vi "SaveTempData.vi"(2 "temp data":dbl[][][](array[numeric]), 3 "Exp_params":T3={"filename"="201612011532", "ExpFilePath"=path "\\\\10.0.0.7\\takada2/DATA/HBT6/data/Test/201612011532.h5", "File Ref list"=[16777216, 33554432], "sweep_dim"=[4, 2], "sweep_list"=[], "readout_list"=["ADC0", "ADC1"], "Sweep instrument bools"=[[0, 0], [0, 0], [0, 0], [0, 0], [0, 0], [0, 0], [0, 0], [0, 0], [0, 0], [0, 0], [0, 0], [0, 0], [0, 0], [0, 0], [0, 0], [0, 0], [0, 0], [0, 0], [0, 0], [0, 0], [0, 0], [0, 0], [0, 0], [0, 0], [0, 0], [0, 0], [0, 0], [0, 0], [0, 0], [0, 0], [0, 0]], "Read out instrument bools"=[[1, 0]], "Experimental bool list"=[FALSE, TRUE], "Initial move"=[{"Name"="None", "kind"=100, "Value"=0.0}], "FPGA Ref"=refnum, "Inst_parameters"={"ConfigFilePath"=path "\\\\10.0.0.7\\takada2/DATA/HBT6/data/Configs/HBT6_ramp_1.h5", "Inst_list"=["ADC", "AWG", "Freq", "Power", "sus", "rus", "rls", "sls", "suq", "suu", "sur", "suc", "sul", "ruq", "ruu", "rur", "ruc", "rul", "rlq", "rlu", "rlr", "rlc", "rll", "slq", "slu", "slr", "slc", "sll", "tu", "t", "tl", "fast_sequence"], "fast_mode"=[1, 1], "Wait_times"=[1, 1, 1, 1], "Inst_array"=[{"Kind"=0, "Strings"=["ADC", "", "V", "ADC0;ADC1", "V;V", "1.0;1.0"], "uint64s"=[10, 2, 250000, 0, 100, 10106, 1000000, 1, 0, 1], "Doubles"=[1.0], "DAQmx take out list"=[]}, {"Kind"=7, "Strings"=["AWG", "10.0.0.4", "", "C:\\Documents and Settings\\Bauerle\\Mes documents\\Bautze\\FPGA-clean_works_1.13.6_batchtest\\Python\\AWG", "dummy", "SAWnstrig_v4.py"], "uint64s"=[2, 0, 0, 3, 0, 0, 0, 0, 0, 0, 0, 0, 0, 0], "Doubles"=[1200000000.0, 1.0, 0.0, 1.0, 0.0, 1.0, 0.0, 1.0, 0.0, 1.0, 0.0, 1.0, 0.0], "DAQmx take out list"=[]}, {"Kind"=6, "Strings"=["Freq", "0:19", "GHz"], "uint64s"=[1, 0, 0, 0, 2, 0, 0, 0], "Doubles"=[2.0, -30.0, 200.0, 100.0, 0.0, 6.000999927520752, 9.000000318337698e-06, 30.0, -145.0], "DAQmx take out list"=[]}, {"Kind"=6, "Strings"=["Power", "0:19", "GHz"], "uint64s"=[1, 0, 1, 0, 2, 0, 0, 0], "Doubles"=[2.0, -30.0, 200.0, 100.0, 0.0, 6.000999927520752, 9.000000318337698e-06, 30.0, -145.0], "DAQmx take out list"=[]}, {"Kind"=4, "Strings"=["sus", "10.0.0.2", "mV"], "uint64s"=[0, 1], "Doubles"=[1.0, -1.0, 1.0, -1.0, 1.0], "DAQmx take out list"=[]}, {"Kind"=4, "Strings"=["rus", "10.0.0.2", "mV"], "uint64s"=[0, 2], "Doubles"=[1.0, -1.0, 1.0, -1.0, 1.0], "DAQmx take out list"=[]}, {"Kind"=4, "Strings"=["rls", "10.0.0.2", "mV"], "uint64s"=[0, 3], "Doubles"=[1.0, -1.0, 1.0, -1.0, 1.0], "DAQmx take out list"=[]}, {"Kind"=4, "Strings"=["sls", "10.0.0.2", "mV"], "uint64s"=[0, 4], "Doubles"=[1.0, -1.0, 1.0, -1.0, 1.0], "DAQmx take out list"=[]}, {"Kind"=4, "Strings"=["suq", "10.0.0.2", "V"], "uint64s"=[0, 5], "Doubles"=[0.30000001192092896, -2.0, 1.0, -1.0, 1.0], "DAQmx take out list"=[]}, {"Kind"=4, "Strings"=["suu", "10.0.0.2", "V"], "uint64s"=[0, 6], "Doubles"=[0.30000001192092896, -2.0, 1.0, -1.0, 1.0], "DAQmx take out list"=[]}, {"Kind"=4, "Strings"=["sur", "10.0.0.2", "V"], "uint64s"=[0, 7], "Doubles"=[0.30000001192092896, -2.0, 1.0, -1.0, 1.0], "DAQmx take out list"=[]}, {"Kind"=4, "Strings"=["suc", "10.0.0.2", "V"], "uint64s"=[1, 0], "Doubles"=[0.30000001192092896, -2.0, 1.0, -1.0, 1.0], "DAQmx take out list"=[]}, {"Kind"=4, "Strings"=["sul", "10.0.0.2", "V"], "uint64s"=[1, 1], "Doubles"=[0.30000001192092896, -2.0, 1.0, -1.0, 1.0], "DAQmx take out list"=[]}, {"Kind"=4, "Strings"=["ruq", "10.0.0.2", "V"], "uint64s"=[1, 2], "Doubles"=[0.30000001192092896, -2.0, 1.0, -1.0, 1.0], "DAQmx take out list"=[]}, {"Kind"=4, "Strings"=["ruu", "10.0.0.2", "V"], "uint64s"=[1, 3], "Doubles"=[0.30000001192092896, -2.0, 1.0, -1.0, 1.0], "DAQmx take out list"=[]}, {"Kind"=4, "Strings"=["rur", "10.0.0.2", "V"], "uint64s"=[1, 5], "Doubles"=[0.30000001192092896, -2.0, 1.0, -1.0, 1.0], "DAQmx take out list"=[]}, {"Kind"=4, "Strings"=["ruc", "10.0.0.2", "V"], "uint64s"=[1, 6], "Doubles"=[0.30000001192092896, -2.0, 1.0, -1.0, 1.0], "DAQmx take out list"=[]}, {"Kind"=4, "Strings"=["rul", "10.0.0.2", "V"], "uint64s"=[1, 7], "Doubles"=[0.30000001192092896, -2.0, 1.0, -1.0, 1.0], "DAQmx take out list"=[]}, {"Kind"=4, "Strings"=["rlq", "10.0.0.2", "V"], "uint64s"=[2, 0], "Doubles"=[0.30000001192092896, -2.0, 1.0, -1.0, 1.0], "DAQmx take out list"=[]}, {"Kind"=4, "Strings"=["rlu", "10.0.0.2", "V"], "uint64s"=[2, 1], "Doubles"=[0.30000001192092896, -2.0, 1.0, -1.0, 1.0], "DAQmx take out list"=[]}, {"Kind"=4, "Strings"=["rlr", "10.0.0.2", "V"], "uint64s"=[2, 2], "Doubles"=[0.30000001192092896, -2.0, 1.0, -1.0, 1.0], "DAQmx take out list"=[]}, {"Kind"=4, "Strings"=["rlc", "10.0.0.2", "V"], "uint64s"=[2, 3], "Doubles"=[0.30000001192092896, -2.0, 1.0, -1.0, 1.0], "DAQmx take out list"=[]}, {"Kind"=4, "Strings"=["rll", "10.0.0.2", "V"], "uint64s"=[2, 4], "Doubles"=[0.30000001192092896, -2.0, 1.0, -1.0, 1.0], "DAQmx take out list"=[]}, {"Kind"=4, "Strings"=["slq", "10.0.0.2", "V"], "uint64s"=[2, 5], "Doubles"=[0.30000001192092896, -2.0, 1.0, -1.0, 1.0], "DAQmx take out list"=[]}, {"Kind"=4, "Strings"=["slu", "10.0.0.2", "V"], "uint64s"=[2, 6], "Doubles"=[0.30000001192092896, -2.0, 1.0, -1.0, 1.0], "DAQmx take out list"=[]}, {"Kind"=4, "Strings"=["slr", "10.0.0.2", "V"], "uint64s"=[2, 7], "Doubles"=[0.30000001192092896, -2.0, 1.0, -1.0, 1.0], "DAQmx take out list"=[]}, {"Kind"=4, "Strings"=["slc", "10.0.0.2", "V"], "uint64s"=[3, 0], "Doubles"=[0.30000001192092896, -2.0, 1.0, -1.0, 1.0], "DAQmx take out list"=[]}, {"Kind"=4, "Strings"=["sll", "10.0.0.2", "V"], "uint64s"=[3, 1], "Doubles"=[0.30000001192092896, -2.0, 1.0, -1.0, 1.0], "DAQmx take out list"=[]}, {"Kind"=4, "Strings"=["tu", "10.0.0.2", "V"], "uint64s"=[3, 2], "Doubles"=[0.30000001192092896, -2.0, 1.0, -1.0, 1.0], "DAQmx take out list"=[]}, {"Kind"=4, "Strings"=["t", "10.0.0.2", "V"], "uint64s"=[3, 3], "Doubles"=[0.30000001192092896, -2.0, 1.0, -1.0, 1.0], "DAQmx take out list"=[]}, {"Kind"=4, "Strings"=["tl", "10.0.0.2", "V"], "uint64s"=[3, 4], "Doubles"=[0.30000001192092896, -2.0, 1.0, -1.0, 1.0], "DAQmx take out list"=[]}, {"Kind"=9, "Strings"=["fast_sequence", "10.0.0.2", "V"], "uint64s"=[6661, 300, 200, 0, 0, 1, 2, 3, 4, 5, 6, 7, 16, 17, 18, 19, 20, 21, 22, 23, 0], "Doubles"=[0.5, -0.5, -1.0, -1.0], "DAQmx take out list"=[]}]}} {"File Ref list" format="%.0x"}, 4 "count":i32) -> (0 "count out":i32, 1 "Exp_params out":T3 {"File Ref list" format="%.0x"})   [LabVIEW 2010]
uses:
  <vilib>/addons/h5labview2/base/hid_t.ctl
  fpga-bitfile-ref.ctl
  <vilib>/addons/h5labview2/dataset/H5Dwrite.llb/H5Dwrite.xnode
  <vilib>/addons/h5labview2/base/lib_path.vi
  <vilib>/addons/h5labview2/base/H5Equery.vi
  <vilib>/addons/h5labview2/dataset/H5D.lvlib
  <vilib>/addons/h5labview2/space/H5S.lvlib
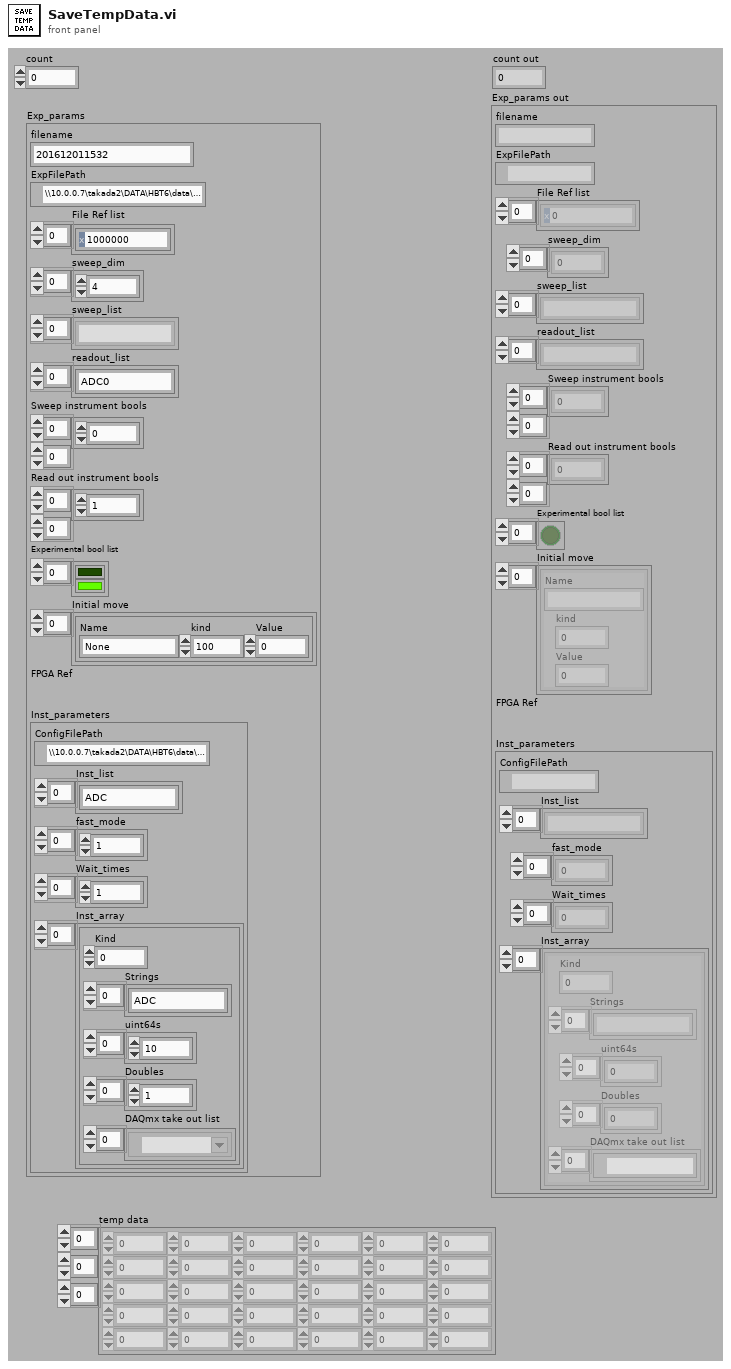
[diagram p1: front panel]
types:
  T1 = typedef "hid_t.ctl" = i32
  T2 = typedef "fpga-bitfile-ref.ctl" = refnum<k20>
  T3 = cluster{"filename":string, "ExpFilePath":path, "File Ref list":T1[], "sweep_dim":u64[], "sweep_list":string[], "readout_list":string[], "Sweep instrument bools":u64[][], "Read out instrument bools":u64[][], "Experimental bool list":bool[], "Initial move":cluster{"Name":string, "kind":u64, "Value":dbl}[], "FPGA Ref":T2, "Inst_parameters":cluster{"ConfigFilePath":path, "Inst_list":string[], "fast_mode":u8[], "Wait_times":u64[], "Inst_array":cluster{"Kind":u16, "Strings":string[], "uint64s":u64[], "Doubles":dbl[], "DAQmx take out list":refnum<k21>[]}[]}}
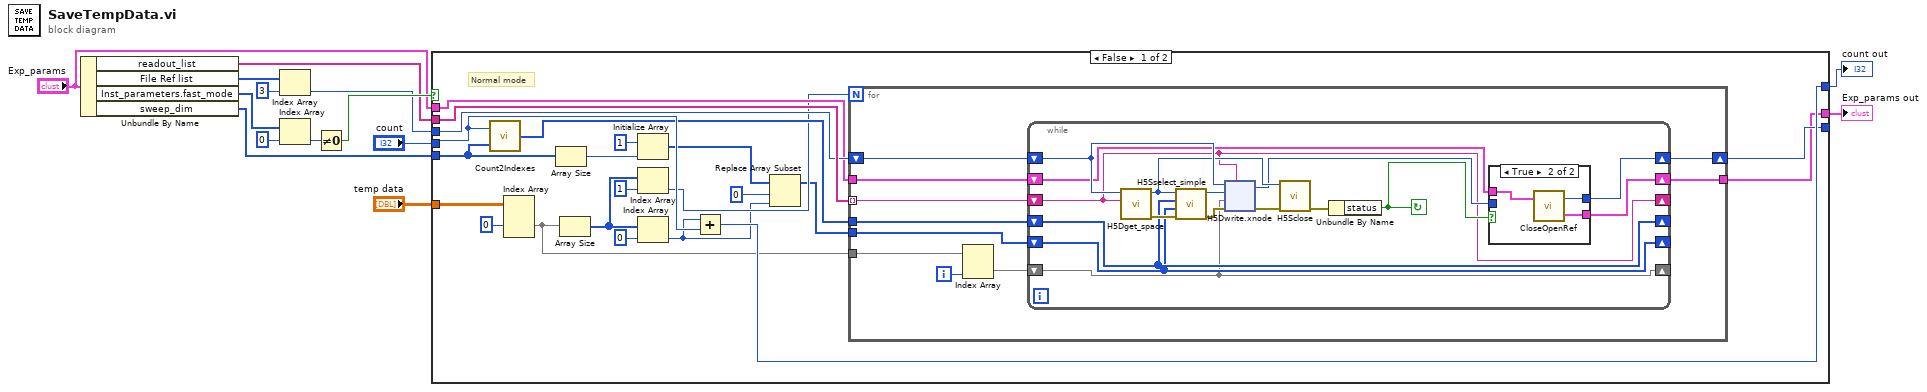
[diagram p0: block diagram]
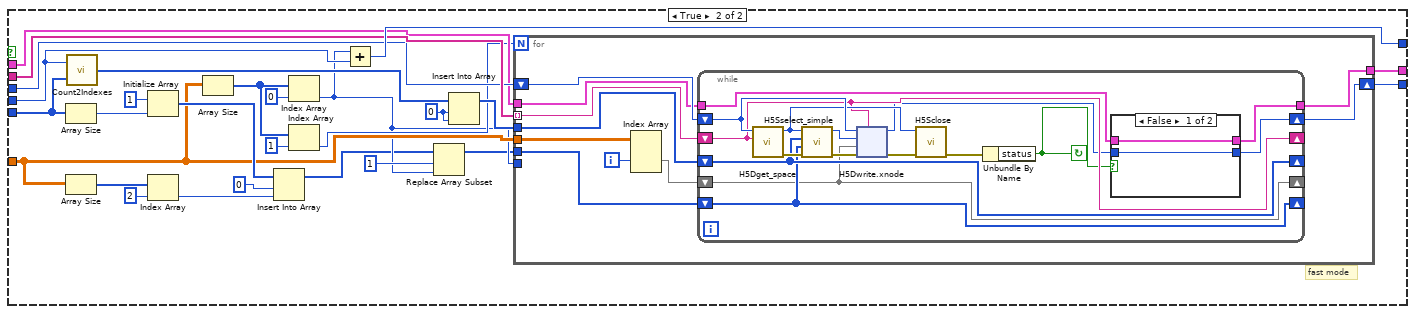
[diagram p3: hidden frame]
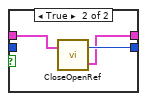
[diagram p4: hidden frame]
diagram:
  n1 = Unbundle By Name("Exp_params") -> ("readout_list"=w8:string[], "File Ref list"=w3:T1[], "Inst_parameters.fast_mode"=w12:u8[], "sweep_dim"=w7:u64[])
  n2 = Index Array(array=w3, index=3) -> (element=w5:T1)
  n3 = Index Array(array=w12, index=0) -> (element=w10:u8)
  n4 = Not Equal To 0?(x=w10) -> (x != 0?=w9:bool)
  n5 = case shown="False" w9 {
    tunnel: w8 -> [w34 w106]
    tunnel: w5 -> [w31 w105]
    tunnel: w7 -> [w21 w108]
    tunnel: "count" -> [w33 w100]
    tunnel: [w32 w107] -> w13
    tunnel: [w30 w104] -> _
    tunnel: "temp data" -> [w36 w94]
    tunnel: "Exp_params" -> [w29 w99]
    tunnel: [w28 w98] -> w1
    frame False {
      # "Normal mode"
      n6 = call "Count2Indexes.vi"("sweep_dim"=w21, "Count"=w33) -> ("Indexes"=w27:u64[])
      n7 = Index Array(array=w36, index (dim 1)=0) -> (element=w26:dbl[][])  [unwired: 2 in]
      n8 = Array Size(array=w21) -> (size(s)=w20:i32)
      n9 = Array Size(array=w26) -> (size(s)=w23:i32[])
      n10 = Initialize Array(1, w20) -> (w18:i32[])
      n11 = Index Array(array=w23, index=1) -> (element=w24:i32)
      n12 = Index Array(array=w23, index=0) -> (element=w15:i32)
      n13 = Add(x=w15, y=w33) -> (x+y=w32:i32)
      n14 = Replace Array Subset(array=w18, new element=w15, index=0) -> (w17:i32[])
      n15 = for {
        N: w24 -> [_]
        shift-right: [w43] -> w30
        shift-left: w31 -> [w46]
        tunnel: w34 -> [w45] mode=indexing
        tunnel: w27 -> [w44]
        tunnel: w26 -> [w40]
        tunnel: w29 -> [w42]
        tunnel: [w41] -> w28
        tunnel: w17 -> [w37]
        i -> [w38]
        n16 = Index Array(array=w40, index (col)=w38) -> (element=w39:dbl[])  [unwired: 1 in]
        n17 = while {
          shift-right: [w54] -> w43
          shift-left: w46 -> [w60]
          shift-right: [w52] -> w41
          shift-left: w42 -> [w53]
          shift-right: [w47] -> _
          shift-left: w39 -> [w47]
          shift-right: [w49] -> _
          shift-left: w44 -> [w49]
          shift-right: [w48] -> _
          shift-left: w37 -> [w48]
          shift-right: [w50] -> _
          shift-left: w45 -> [w50]
          stop <- w51 continue-if-true
          n18 = call <vilib>:"H5Dget_space.vi"("obj (.)"=w50, "ref in"=w60) -> ("error out"=w62:errorcluster, "space out"=w58:T1)  [unwired: 8 in]
          n19 = call <vilib>:"H5Sselect_simple.vi"("error in (no error)"=w62, "count"=w48, "start"=w49, "space in"=w58) -> ("error out"=w61:errorcluster, "space out"=w59:T1)  [unwired: 6 in]
          n20 = xnode "H5Dwrite.xnode"("dataset name"=w50, "error in (no error)"=w61, "data"=w47, "file space"=w59, "ref in"=w60) -> ("error out"=w57:errorcluster, "ref out"=w55:i32)  [unwired: 2 in, 1 out]
          n21 = call <vilib>:"H5Sclose.vi"("error in (no error)"=w57, "space in"=w58) -> ("error out"=w56:errorcluster)  [unwired: 9 in]
          n22 = Unbundle By Name(w56) -> ("status"=w51:bool)
          n23 = case shown="True" w51 {
            tunnel: w55 -> [w64 _]
            tunnel: [w64 w66] -> w54
            tunnel: w53 -> [w63 w67]
            tunnel: [w63 w65] -> w52
            frame False {
            }
            frame True {
              n24 = call "CloseOpenRef.vi"("Exp_params"=w67) -> ("Exp_params_out"=w65:T3, "group out"=w66:T1)  [unwired: 1 in]
            }
          }
        }
      }
    }
    frame True {
      w97 = 0
      # "fast mode"
      n25 = Array Size(array=w108) -> (size(s)=w110:i32)
      n26 = Array Size(array=w94) -> (size(s)=w103:i32[])
      n27 = call "Count2Indexes.vi"("sweep_dim"=w108, "Count"=w100) -> ("Indexes"=w96:u64[])
      n28 = Initialize Array(u32 1, w110) -> (w111:u32[])
      n29 = Index Array(array=w103, index=2) -> (element=w101:i32)
      n30 = Array Size(array=w94) -> (size(s)=w91:i32[])
      n31 = Insert Into Array(array=w111, index=0, new element=w101) -> (w87:u32[])
      n32 = Index Array(array=w91, index=0) -> (element=w88:i32)
      n33 = Index Array(array=w91, index=1) -> (element=w92:i32)
      n34 = Add(x=w88, y=w100) -> (x+y=w107:i32)
      n35 = Replace Array Subset(array=w87, new element=w88, index=1) -> (w86:u32[])
      n36 = Insert Into Array(array=w96, index=w97, new element=w97) -> (w95:u64[])
      n37 = for {
        N: w92 -> [_]
        tunnel: w94 -> [w116]
        tunnel: w106 -> [w122] mode=indexing
        tunnel: w95 -> [w120]
        shift-right: [w119] -> w104
        shift-left: w105 -> [w121]
        tunnel: w99 -> [w118]
        tunnel: [w117] -> w98
        tunnel: w88 -> [_]
        tunnel: w86 -> [w113]
        i -> [w114]
        n38 = Index Array(array=w116, index (dim 1)=w114) -> (element=w115:dbl[][])  [unwired: 2 in]
        n39 = while {
          shift-right: [w128] -> _
          shift-left: w115 -> [w128]
          shift-right: [w129] -> _
          shift-left: w113 -> [w129]
          shift-right: [w130] -> _
          shift-left: w120 -> [w130]
          shift-right: [w131] -> _
          shift-left: w122 -> [w131]
          shift-right: [w123] -> w119
          shift-left: w121 -> [w138]
          tunnel: w118 -> [w127]
          tunnel: [w125] -> w117
          stop <- w126 continue-if-true
          n40 = call <vilib>:"H5Dget_space.vi"("obj (.)"=w131, "ref in"=w138) -> ("error out"=w137:errorcluster, "space out"=w135:T1)  [unwired: 8 in]
          n41 = call <vilib>:"H5Sselect_simple.vi"("error in (no error)"=w137, "count"=w129, "start"=w130, "space in"=w135) -> ("error out"=w136:errorcluster, "space out"=w134:T1)  [unwired: 6 in]
          n42 = xnode "H5Dwrite.xnode"("dataset name"=w131, "error in (no error)"=w136, "data"=w128, "file space"=w134, "ref in"=w138) -> ("error out"=w133:errorcluster, "ref out"=w124:T1)  [unwired: 2 in, 1 out]
          n43 = call <vilib>:"H5Sclose.vi"("error in (no error)"=w133, "space in"=w135) -> ("error out"=w132:errorcluster)  [unwired: 9 in]
          n44 = Unbundle By Name(w132) -> ("status"=w126:bool)
          n45 = case shown="False" w126 {
            tunnel: w127 -> [w140 w143]
            tunnel: [w140 w141] -> w125
            tunnel: w124 -> [w139 _]
            tunnel: [w139 w142] -> w123
            frame False {
            }
            frame True {
              n46 = call "CloseOpenRef.vi"("Exp_params"=w143) -> ("Exp_params_out"=w141:T3, "group out"=w142:T1)  [unwired: 1 in]
            }
          }
        }
      }
    }
  }
  "count out" <- w13
  "Exp_params out" <- w1
